vi "ReadRawRasnik.vi"(3 "Lines":string[](array[string])) -> (0 "X cluster":string[](array[string]), 1 "Y cluster":string[](array[string]), 2 "angle cluster":string[](array[string]))   [LabVIEW 2015]
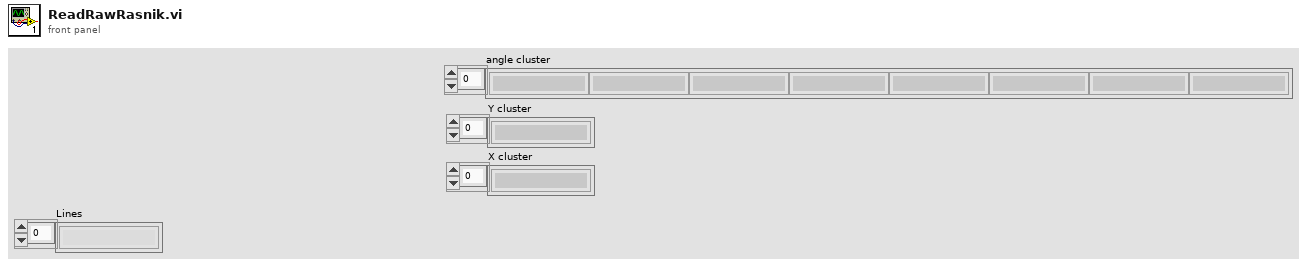
[diagram p1: front panel]
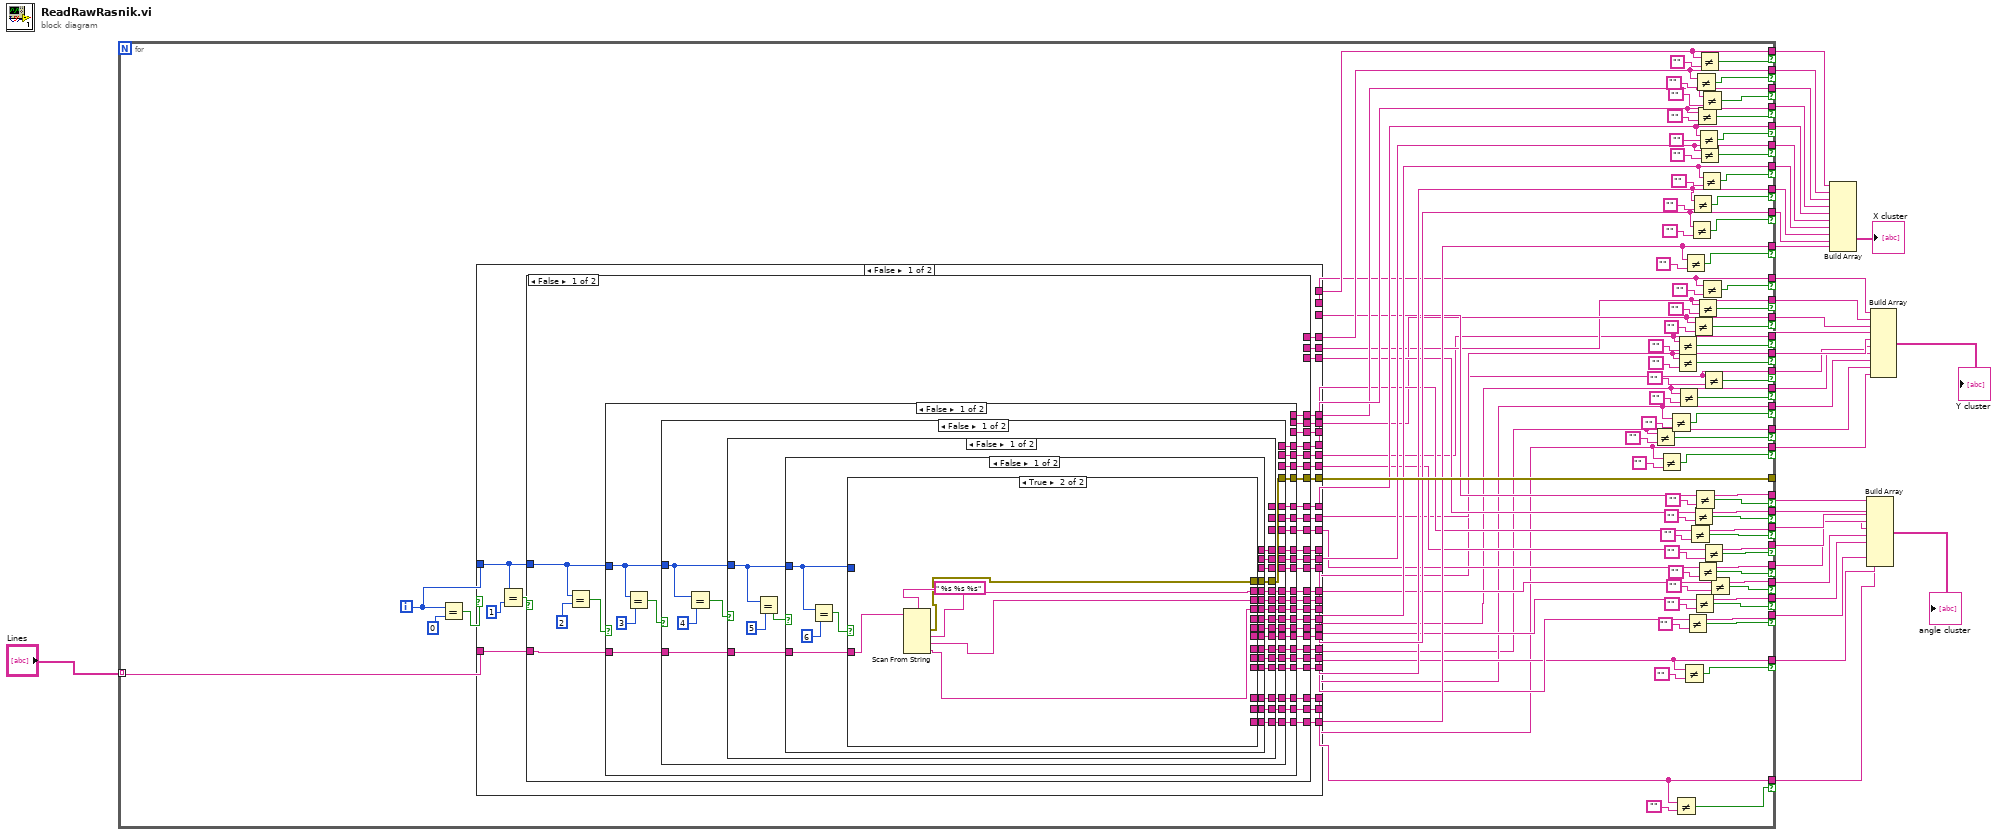
[diagram p0: block diagram]
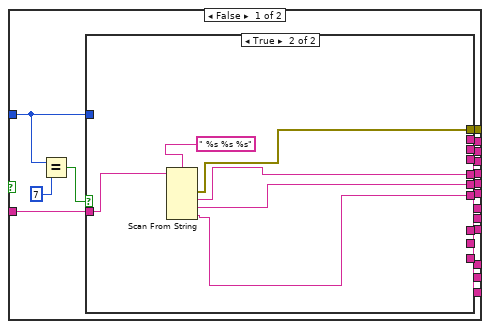
[diagram p2: hidden frame]
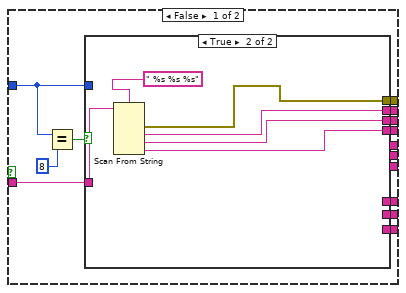
[diagram p3: hidden frame]
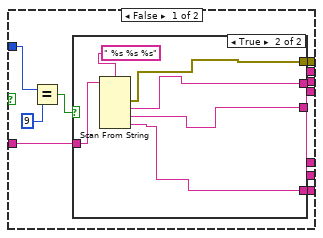
[diagram p4: hidden frame]
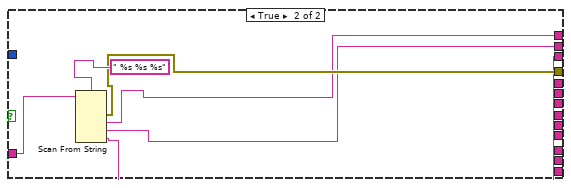
[diagram p6: hidden frame]
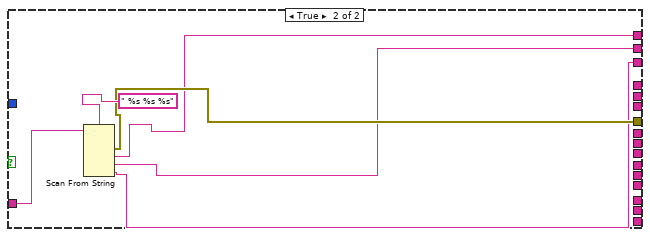
[diagram p7: hidden frame]
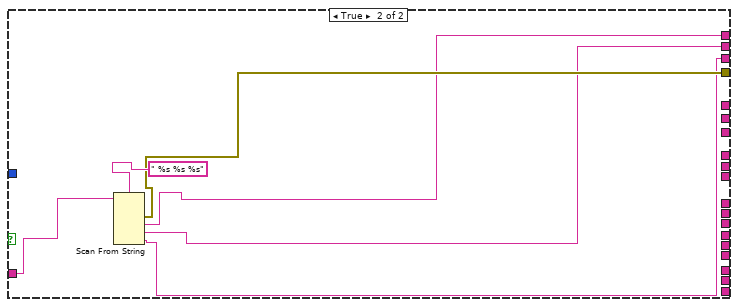
[diagram p8: hidden frame]
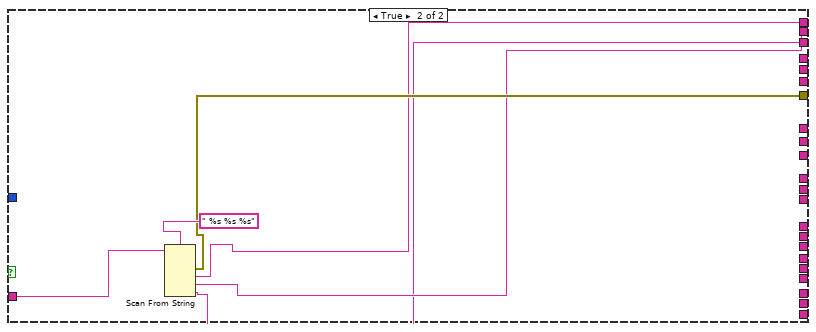
[diagram p9: hidden frame]
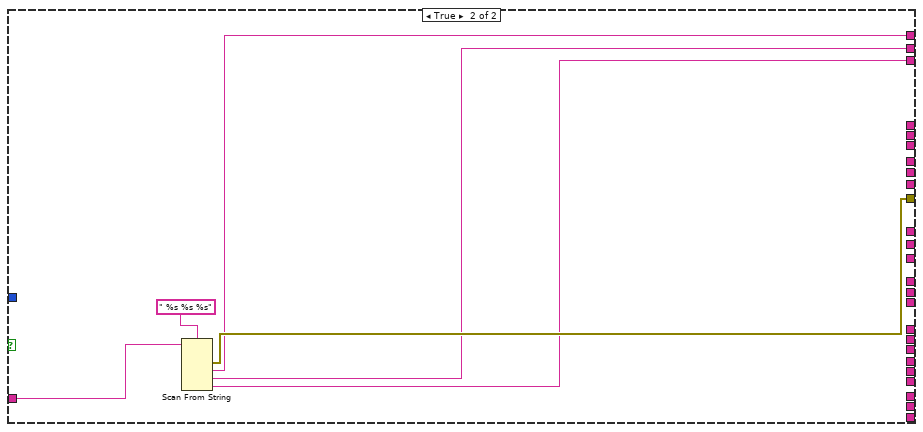
[diagram p10: hidden frame]
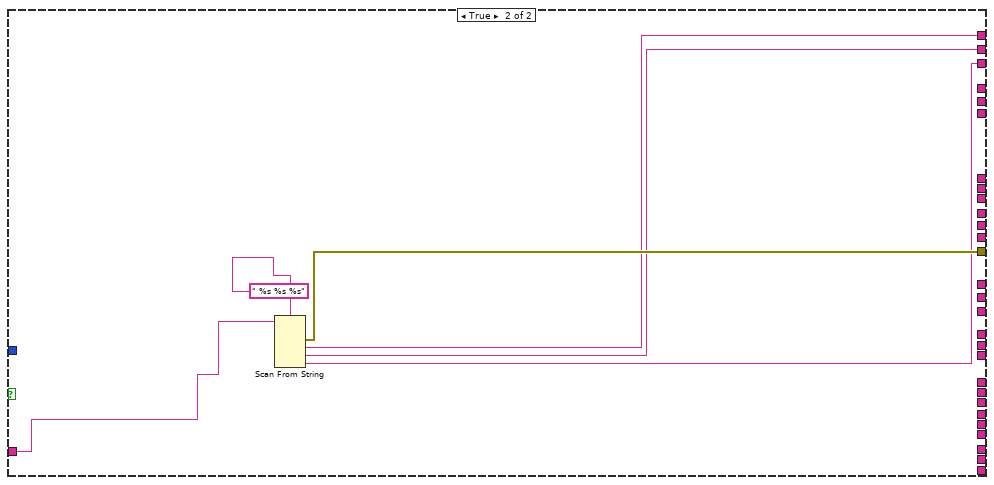
[diagram p11: hidden frame]
diagram:
  n1 = for {
    tunnel: "Lines" -> [w126] mode=indexing
    tunnel: [w125] -> _
    tunnel: [w122] -> w33 if=w123
    tunnel: [w112] -> w32 if=w111
    tunnel: [w95] -> w31 if=w110
    tunnel: [w96] -> w30 if=w109
    tunnel: [w97] -> w29 if=w108
    tunnel: [w98] -> w28 if=w107
    tunnel: [w99] -> w27 if=w106
    tunnel: [w100] -> w26 if=w105
    tunnel: [w101] -> w25 if=w104
    tunnel: [w59] -> w22 if=w58
    tunnel: [w60] -> w21 if=w57
    tunnel: [w61] -> w20 if=w56
    tunnel: [w48] -> w19 if=w35
    tunnel: [w47] -> w18 if=w36
    tunnel: [w46] -> w17 if=w37
    tunnel: [w45] -> w16 if=w38
    tunnel: [w44] -> w15 if=w39
    tunnel: [w43] -> w14 if=w40
    tunnel: [w42] -> w13 if=w41
    tunnel: [w102] -> w12 if=w103
    tunnel: [w76] -> w1 if=w77
    tunnel: [w75] -> w10 if=w78
    tunnel: [w74] -> w9 if=w79
    tunnel: [w73] -> w8 if=w80
    tunnel: [w72] -> w7 if=w81
    tunnel: [w71] -> w6 if=w82
    tunnel: [w70] -> w5 if=w83
    tunnel: [w69] -> w4 if=w84
    tunnel: [w68] -> w3 if=w85
    tunnel: [w65] -> w2 if=w66
    i -> [w128]
    n2 = Equal?(x=w128, y=0) -> (x = y?=w127:bool)
    n3 = case shown="False" w127 {
      tunnel: w126 -> [w160 w368]
      tunnel: w128 -> [w158 _]
      tunnel: [w157 w367] -> w125
      tunnel: [w156 _] -> w65
      tunnel: [w155 _] -> w42
      tunnel: [w154 _] -> w102
      tunnel: [w153 _] -> w101
      tunnel: [w152 _] -> w43
      tunnel: [w151 _] -> w68
      tunnel: [w150 _] -> w100
      tunnel: [w149 _] -> w44
      tunnel: [w148 _] -> w69
      tunnel: [w147 _] -> w98
      tunnel: [w146 _] -> w46
      tunnel: [w145 _] -> w71
      tunnel: [w144 _] -> w72
      tunnel: [w143 _] -> w47
      tunnel: [w142 _] -> w97
      tunnel: [w141 _] -> w96
      tunnel: [w140 _] -> w48
      tunnel: [w139 _] -> w73
      tunnel: [w138 _] -> w95
      tunnel: [w137 _] -> w61
      tunnel: [w136 _] -> w74
      tunnel: [w135 _] -> w112
      tunnel: [w134 _] -> w60
      tunnel: [w133 _] -> w75
      tunnel: [_ w366] -> w122
      tunnel: [_ w365] -> w59
      tunnel: [_ w364] -> w76
      tunnel: [w132 _] -> w99
      tunnel: [w131 _] -> w45
      tunnel: [w130 _] -> w70
      frame False {
        n4 = Equal?(x=w158, y=1) -> (x = y?=w161:bool)
        n5 = case shown="False" w161 {
          tunnel: w160 -> [w189 w362]
          tunnel: w158 -> [w187 _]
          tunnel: [w186 w361] -> w157
          tunnel: [w185 _] -> w156
          tunnel: [w184 _] -> w155
          tunnel: [w183 _] -> w154
          tunnel: [w182 _] -> w153
          tunnel: [w181 _] -> w152
          tunnel: [w180 _] -> w151
          tunnel: [w179 _] -> w150
          tunnel: [w178 _] -> w149
          tunnel: [w177 _] -> w148
          tunnel: [w176 _] -> w147
          tunnel: [w175 _] -> w146
          tunnel: [w174 _] -> w145
          tunnel: [w173 _] -> w144
          tunnel: [w172 _] -> w143
          tunnel: [w171 _] -> w142
          tunnel: [w170 _] -> w141
          tunnel: [w169 _] -> w140
          tunnel: [w168 _] -> w139
          tunnel: [w167 _] -> w138
          tunnel: [w166 _] -> w137
          tunnel: [w165 _] -> w136
          tunnel: [_ w360] -> w135
          tunnel: [_ w359] -> w134
          tunnel: [_ w358] -> w133
          tunnel: [w164 _] -> w132
          tunnel: [w163 _] -> w131
          tunnel: [w162 _] -> w130
          frame False {
            n6 = Equal?(x=w187, y=2) -> (x = y?=w190:bool)
            n7 = case shown="False" w190 {
              tunnel: w189 -> [w214 w356]
              tunnel: w187 -> [w213 _]
              tunnel: [w212 w355] -> w186
              tunnel: [w211 _] -> w185
              tunnel: [w210 _] -> w184
              tunnel: [w209 _] -> w183
              tunnel: [w208 _] -> w182
              tunnel: [w207 _] -> w181
              tunnel: [w206 _] -> w180
              tunnel: [w205 _] -> w179
              tunnel: [w204 _] -> w178
              tunnel: [w203 _] -> w177
              tunnel: [w202 _] -> w176
              tunnel: [w201 _] -> w175
              tunnel: [w200 _] -> w174
              tunnel: [w199 _] -> w173
              tunnel: [w198 _] -> w172
              tunnel: [w197 _] -> w171
              tunnel: [w196 _] -> w170
              tunnel: [w195 _] -> w169
              tunnel: [w194 _] -> w168
              tunnel: [_ w354] -> w167
              tunnel: [_ w353] -> w166
              tunnel: [_ w352] -> w165
              tunnel: [w193 _] -> w164
              tunnel: [w192 _] -> w163
              tunnel: [w191 _] -> w162
              frame False {
                n8 = Equal?(x=w213, y=3) -> (x = y?=w215:bool)
                n9 = case shown="False" w215 {
                  tunnel: w214 -> [w237 w350]
                  tunnel: w213 -> [w236 _]
                  tunnel: [w235 w349] -> w212
                  tunnel: [w234 _] -> w211
                  tunnel: [w233 _] -> w210
                  tunnel: [w232 _] -> w209
                  tunnel: [w231 _] -> w208
                  tunnel: [w230 _] -> w207
                  tunnel: [w229 _] -> w206
                  tunnel: [w228 _] -> w205
                  tunnel: [w227 _] -> w204
                  tunnel: [w226 _] -> w203
                  tunnel: [w225 _] -> w202
                  tunnel: [w224 _] -> w201
                  tunnel: [w223 _] -> w200
                  tunnel: [w222 _] -> w199
                  tunnel: [w221 _] -> w198
                  tunnel: [w220 _] -> w197
                  tunnel: [_ w348] -> w196
                  tunnel: [_ w347] -> w195
                  tunnel: [_ w346] -> w194
                  tunnel: [w219 _] -> w193
                  tunnel: [w218 _] -> w192
                  tunnel: [w217 _] -> w191
                  frame False {
                    n10 = Equal?(x=w236, y=4) -> (x = y?=w238:bool)
                    n11 = case shown="False" w238 {
                      tunnel: w237 -> [w257 w344]
                      tunnel: w236 -> [w256 _]
                      tunnel: [w255 w343] -> w235
                      tunnel: [w254 _] -> w234
                      tunnel: [w253 _] -> w233
                      tunnel: [w252 _] -> w232
                      tunnel: [w251 _] -> w231
                      tunnel: [w250 _] -> w230
                      tunnel: [w249 _] -> w229
                      tunnel: [w248 _] -> w228
                      tunnel: [w247 _] -> w227
                      tunnel: [w246 _] -> w226
                      tunnel: [w245 _] -> w225
                      tunnel: [w244 _] -> w224
                      tunnel: [w243 _] -> w223
                      tunnel: [_ w342] -> w222
                      tunnel: [_ w341] -> w221
                      tunnel: [_ w340] -> w220
                      tunnel: [w242 _] -> w219
                      tunnel: [w241 _] -> w218
                      tunnel: [w240 _] -> w217
                      frame False {
                        n12 = Equal?(x=w256, y=5) -> (x = y?=w258:bool)
                        n13 = case shown="False" w258 {
                          tunnel: w257 -> [w275 w338]
                          tunnel: w256 -> [w273 _]
                          tunnel: [w272 w337] -> w255
                          tunnel: [w271 _] -> w254
                          tunnel: [w270 _] -> w253
                          tunnel: [w269 _] -> w252
                          tunnel: [w268 _] -> w251
                          tunnel: [w267 _] -> w250
                          tunnel: [w266 _] -> w249
                          tunnel: [w265 _] -> w248
                          tunnel: [w264 _] -> w247
                          tunnel: [w263 _] -> w246
                          tunnel: [_ w336] -> w245
                          tunnel: [_ w335] -> w244
                          tunnel: [_ w334] -> w243
                          tunnel: [w262 _] -> w242
                          tunnel: [w261 _] -> w241
                          tunnel: [w260 _] -> w240
                          frame False {
                            n14 = Equal?(x=w273, y=6) -> (x = y?=w274:bool)
                            n15 = case shown="True" w274 {
                              tunnel: w275 -> [w288 w332]
                              tunnel: w273 -> [w287 _]
                              tunnel: [w286 w331] -> w272
                              tunnel: [w285 _] -> w271
                              tunnel: [w284 _] -> w270
                              tunnel: [w283 _] -> w269
                              tunnel: [w282 _] -> w268
                              tunnel: [w281 _] -> w267
                              tunnel: [w280 _] -> w266
                              tunnel: [w279 _] -> w265
                              tunnel: [w278 _] -> w264
                              tunnel: [w277 _] -> w263
                              tunnel: [_ w330] -> w262
                              tunnel: [_ w329] -> w261
                              tunnel: [_ w328] -> w260
                              frame False {
                                n16 = Equal?(x=w287, y=7) -> (x = y?=w289:bool)
                                n17 = case shown="True" w289 {
                                tunnel: w288 -> [w299 w326]
                                tunnel: w287 -> [w298 _]
                                tunnel: [w297 w325] -> w286
                                tunnel: [w296 _] -> w285
                                tunnel: [w295 _] -> w284
                                tunnel: [w294 _] -> w283
                                tunnel: [w293 _] -> w282
                                tunnel: [w292 _] -> w281
                                tunnel: [w291 _] -> w280
                                tunnel: [_ w324] -> w279
                                tunnel: [_ w323] -> w278
                                tunnel: [_ w322] -> w277
                                frame False {
                                n18 = Equal?(x=w298, y=8) -> (x = y?=w300:bool)
                                n19 = case shown="True" w300 {
                                tunnel: w299 -> [w306 w320]
                                tunnel: w298 -> [w307 _]
                                tunnel: [w305 w319] -> w297
                                tunnel: [w304 _] -> w296
                                tunnel: [w303 _] -> w295
                                tunnel: [w302 _] -> w294
                                tunnel: [_ w318] -> w293
                                tunnel: [_ w317] -> w292
                                tunnel: [_ w316] -> w291
                                frame False {
                                n20 = Equal?(x=w307, y=9) -> (x = y?=w308:bool)
                                n21 = case shown="True" w308 {
                                tunnel: w306 -> [_ w314]
                                tunnel: [_ w313] -> w305
                                tunnel: [_ w312] -> w304
                                tunnel: [_ w311] -> w303
                                tunnel: [_ w310] -> w302
                                frame False {
                                }
                                frame True {
                                n22 = Scan From String(format string=" %s %s %s", input string=w314) -> (error out=w313:errorcluster, output 1=w310:string, output 2=w311:string, output 3=w312:string)  [unwired: 5 in, 2 out]
                                }
                                }
                                }
                                frame True {
                                n23 = Scan From String(format string=" %s %s %s", input string=w320) -> (error out=w319:errorcluster, output 1=w318:string, output 2=w317:string, output 3=w316:string)  [unwired: 5 in, 2 out]
                                }
                                }
                                }
                                frame True {
                                n24 = Scan From String(format string=" %s %s %s", input string=w326) -> (error out=w325:errorcluster, output 1=w324:string, output 2=w323:string, output 3=w322:string)  [unwired: 5 in, 2 out]
                                }
                                }
                              }
                              frame True {
                                n25 = Scan From String(format string=" %s %s %s", input string=w332) -> (error out=w331:errorcluster, output 1=w330:string, output 2=w329:string, output 3=w328:string)  [unwired: 5 in, 2 out]
                              }
                            }
                          }
                          frame True {
                            n26 = Scan From String(format string=" %s %s %s", input string=w338) -> (error out=w337:errorcluster, output 1=w336:string, output 2=w335:string, output 3=w334:string)  [unwired: 5 in, 2 out]
                          }
                        }
                      }
                      frame True {
                        n27 = Scan From String(format string=" %s %s %s", input string=w344) -> (error out=w343:errorcluster, output 1=w340:string, output 2=w341:string, output 3=w342:string)  [unwired: 5 in, 2 out]
                      }
                    }
                  }
                  frame True {
                    n28 = Scan From String(format string=" %s %s %s", input string=w350) -> (error out=w349:errorcluster, output 1=w348:string, output 2=w347:string, output 3=w346:string)  [unwired: 5 in, 2 out]
                  }
                }
              }
              frame True {
                n29 = Scan From String(format string=" %s %s %s", input string=w356) -> (error out=w355:errorcluster, output 1=w354:string, output 2=w353:string, output 3=w352:string)  [unwired: 5 in, 2 out]
              }
            }
          }
          frame True {
            n30 = Scan From String(format string=" %s %s %s", input string=w362) -> (error out=w361:errorcluster, output 1=w360:string, output 2=w359:string, output 3=w358:string)  [unwired: 5 in, 2 out]
          }
        }
      }
      frame True {
        n31 = Scan From String(format string=" %s %s %s", input string=w368) -> (error out=w367:errorcluster, output 1=w366:string, output 2=w365:string, output 3=w364:string)  [unwired: 5 in, 2 out]
      }
    }
    n32 = Not Equal?(x=w43, y="") -> (x != y?=w40:bool)
    n33 = Not Equal?(x=w42, y="") -> (x != y?=w41:bool)
    n34 = Not Equal?(x=w44, y="") -> (x != y?=w39:bool)
    n35 = Not Equal?(x=w65, y="") -> (x != y?=w66:bool)
    n36 = Not Equal?(x=w48, y="") -> (x != y?=w35:bool)
    n37 = Not Equal?(x=w47, y="") -> (x != y?=w36:bool)
    n38 = Not Equal?(x=w45, y="") -> (x != y?=w38:bool)
    n39 = Not Equal?(x=w68, y="") -> (x != y?=w85:bool)
    n40 = Not Equal?(x=w102, y="") -> (x != y?=w103:bool)
    n41 = Not Equal?(x=w69, y="") -> (x != y?=w84:bool)
    n42 = Not Equal?(x=w74, y="") -> (x != y?=w79:bool)
    n43 = Not Equal?(x=w101, y="") -> (x != y?=w104:bool)
    n44 = Not Equal?(x=w100, y="") -> (x != y?=w105:bool)
    n45 = Not Equal?(x=w61, y="") -> (x != y?=w56:bool)
    n46 = Not Equal?(x=w75, y="") -> (x != y?=w78:bool)
    n47 = Not Equal?(x=w70, y="") -> (x != y?=w83:bool)
    n48 = Not Equal?(x=w76, y="") -> (x != y?=w77:bool)
    n49 = Not Equal?(x=w112, y="") -> (x != y?=w111:bool)
    n50 = Not Equal?(x=w96, y="") -> (x != y?=w109:bool)
    n51 = Not Equal?(x=w60, y="") -> (x != y?=w57:bool)
    n52 = Not Equal?(x=w72, y="") -> (x != y?=w81:bool)
    n53 = Not Equal?(x=w97, y="") -> (x != y?=w108:bool)
    n54 = Not Equal?(x=w122, y="") -> (x != y?=w123:bool)
    n55 = Not Equal?(x=w98, y="") -> (x != y?=w107:bool)
    n56 = Not Equal?(x=w99, y="") -> (x != y?=w106:bool)
    n57 = Not Equal?(x=w95, y="") -> (x != y?=w110:bool)
    n58 = Not Equal?(x=w59, y="") -> (x != y?=w58:bool)
    n59 = Not Equal?(x=w46, y="") -> (x != y?=w37:bool)
    n60 = Not Equal?(x=w73, y="") -> (x != y?=w80:bool)
    n61 = Not Equal?(x=w71, y="") -> (x != y?=w82:bool)
  }
  n62 = Build Array(w33, w32, w31, w30, w29, w28, w27, w26, w25, w12) -> (→"X cluster":string[])
  n63 = Build Array(w1, w10, w9, w8, w7, w6, w5, w4, w3, w2) -> (→"angle cluster":string[])
  n64 = Build Array(w22, w21, w20, w19, w18, w17, w16, w15, w14, w13) -> (→"Y cluster":string[])
